vi "AlazarFFTSetup.vi"(0 "DSP Handle":u64, 1 "Input Channel Mask":u16(ring)=1 items=["CHANNEL_A"=1], 2 "Record Length (samples)":u32, 3 "FFT Length (samples)":u32, 4 "Output Format":u32(ring)=1 items=["U32_AMP2"=0, "U16_LOG"=1, "U16_AMP2"=257, "U8_LOG"=2, "U8_AMP2"=258, "REAL_S32"=3, "IMAG_S32"=4, "FLOAT_AMP2"=10, "FLOAT_LOG"=11, "RAW_PLUS_FFT"=4096], 5 "Footer":u32(ring) items=["FOOTER_NONE", "FOOTER_NPT"], 6 "Reserved":u32, 7 "error in (no error)":errorcluster) -> (20 "DSP Handle":u64, 21 "Bytes Per Output Record":u32, 26 "Return Code":u32, 27 "error out":errorcluster)   [LabVIEW 2009]
uses:
  ATSApi.dll
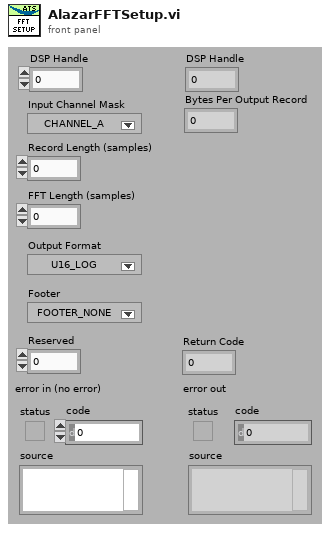
[diagram p1: front panel]
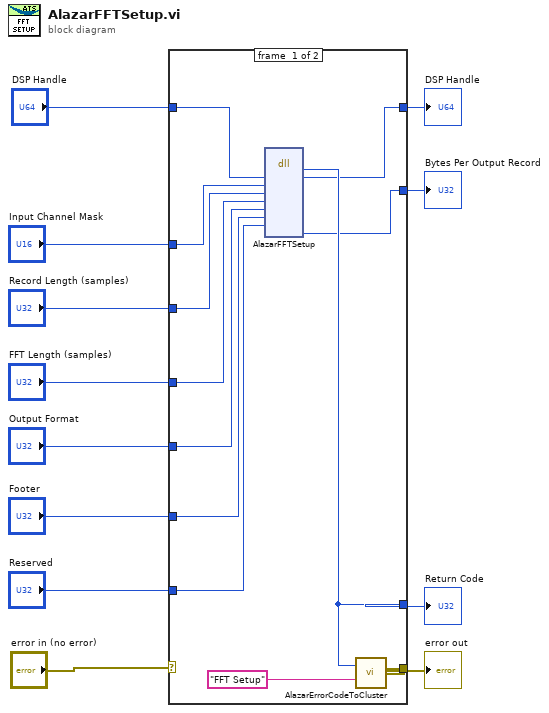
[diagram p0: block diagram]
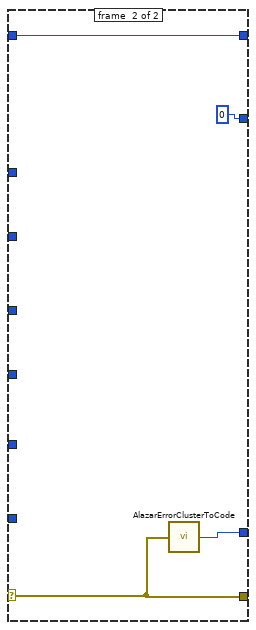
[diagram p2: hidden frame]
diagram:
  n1 = case shown="No Error" "error in (no error)" {
    selector: "error in (no error)" -> [_ w28]
    tunnel: [w21 w28] -> w11
    tunnel: [w23 w27] -> w10
    tunnel: "DSP Handle" -> [w24 w26]
    tunnel: [w20 w26] -> w8
    tunnel: "Input Channel Mask" -> [w19 _]
    tunnel: "Record Length (samples)" -> [w18 _]
    tunnel: "FFT Length (samples)" -> [w17 _]
    tunnel: "Output Format" -> [w16 _]
    tunnel: "Footer" -> [w15 _]
    tunnel: "Reserved" -> [w14 _]
    tunnel: [w13 0] -> w1
    frame #0 {
      n2 = dll-call lib="ATSApi.dll" fn="AlazarFFTSetup"("handle"=w24, "inputChannelMask"=w19, "recordLength_samples"=w18, "fftLength_samples"=w17, "outputFormat"=w16, "footer"=w15, "reserved"=w14) -> ("return type"=w23:u32, "handle"=w20:u64, "bytesPerOutputRecord"=w13:u32)  [unwired: 10 in, 2 out]
      n3 = call "AlazarErrorCodeToCluster.vi"("Message"="FFT Setup", "Error Code"=w23) -> ("error out"=w21:errorcluster)
    }
    frame #1 {
      n4 = call "AlazarErrorClusterToCode.vi"("error in (no error)"=w28) -> ("Error Code"=w27:u32)
    }
  }
  "DSP Handle" <- w8
  "error out" <- w11
  "Return Code" <- w10
  "Bytes Per Output Record" <- w1
